vi "GetControlReferenceInTabControl.vi"(8 "error in (no error)":errorcluster, 10 "Control Name":string, 11 "VI in":refnum<vi>) -> (0 "error out":errorcluster, 2 "Ctl Refnum":refnum<vi>, 3 "VI out":refnum<vi>)   [LabVIEW 2017]
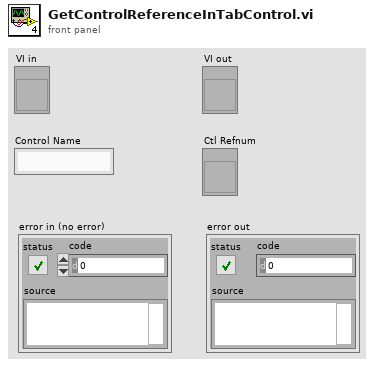
[diagram p1: front panel]
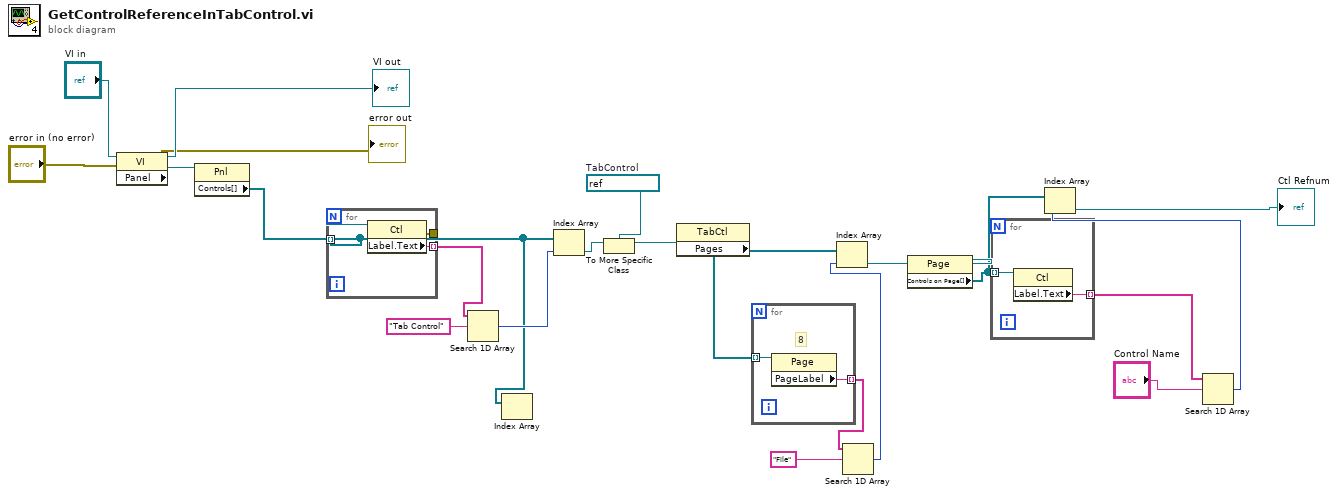
[diagram p0: block diagram]
diagram:
  w1 = refnum<vi> refnum  # TabControl
  n1 = property class="VI"(reference="VI in", error in="error in (no error)") -> (reference out=→"VI out":refnum<vi>, error out=→"error out":errorcluster, "Panel"=w16:refnum<vi>)
  n2 = property class="Pnl"(reference=w16) -> ("Controls[]"=w2:refnum<vi>[])  [unwired: 1 in, 2 out]
  n3 = for {
    tunnel: w2 -> [w25] mode=indexing
    tunnel: [w24] -> w3 mode=indexing
    tunnel: [w23] -> _
    n4 = property class="Ctl"(reference=w25) -> (error out=w23:errorcluster, "Label.Text"=w24:string)  [unwired: 1 in, 1 out]
  }
  n5 = Search 1D Array(1D array=w3, element="Tab Control") -> (index of element=w18:i32)  [unwired: 1 in]
  n6 = Index Array(array=w2) -> ()  [unwired: 1 in, 1 out]
  n7 = Index Array(array=w2, index=w18) -> (element=w4:refnum<vi>)
  n8 = To More Specific Class(target class=w1, reference=w4) -> (specific class reference=w9:refnum<vi>)  [unwired: 1 in, 1 out]
  n9 = property class="TabCtl"(reference=w9) -> ("Pages"=w5:refnum<vi>[])  [unwired: 1 in, 2 out]
  n10 = for {
    tunnel: [w27] -> w7 mode=indexing
    tunnel: w5 -> [w26] mode=indexing
    # "8"
    n11 = property class="Page"(reference=w26) -> ("PageLabel"=w27:string)  [unwired: 1 in, 2 out]
  }
  n12 = Search 1D Array(1D array=w7, element="File") -> (index of element=w6:i32)  [unwired: 1 in]
  n13 = Index Array(array=w5, index=w6) -> (element=w17:refnum<vi>)
  n14 = property class="Page"(reference=w17) -> ("Controls on Page[]"=w12:refnum<vi>[])  [unwired: 1 in, 2 out]
  n15 = for {
    tunnel: [w29] -> w14 mode=indexing
    tunnel: w12 -> [w28] mode=indexing
    n16 = property class="Ctl"(reference=w28) -> ("Label.Text"=w29:string)  [unwired: 1 in, 2 out]
  }
  n17 = Search 1D Array(1D array=w14, element="Control Name") -> (index of element=w11:i32)  [unwired: 1 in]
  n18 = Index Array(array=w12, index=w11) -> (element=→"Ctl Refnum":refnum<vi>)
